vi "Capture.vi"(8 "error in (no error)":errorcluster, 9 "force_length":i8, 10 "capture_channel":u16, 11 "length":i32) -> (0 "error out":errorcluster, 3 "function return":i32)   [LabVIEW 2021, in "vmmsolib.lvlib"]
doc: "DLL_API int WINAPI Capture(int length, unsigned short capture_channel, char force_length);"
uses:
  vmmsolib.lvlib
  vmmso.dll
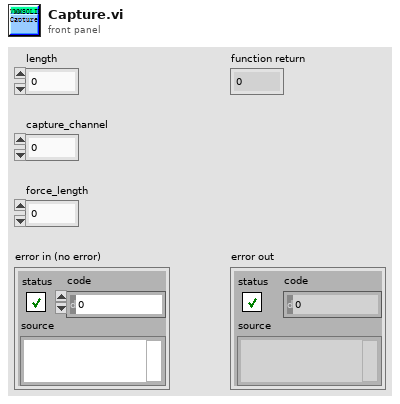
[diagram p1: front panel]
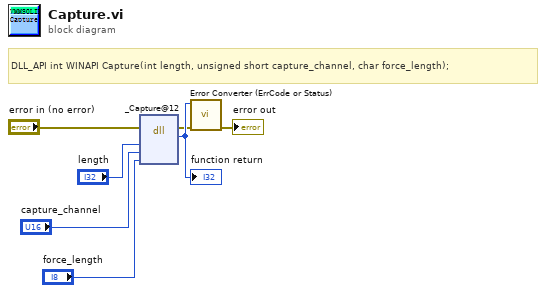
[diagram p0: block diagram]
diagram:
  # "DLL_API int WINAPI Capture(int length, unsigned short capture_channel, char force_length);"
  n1 = dll-call lib="D:/VmMsoSDK/demo-Labview/2021/vmmsolib/vmmso.*" fn="_Capture@12"(error in="error in (no error)", "length"="length", "capture_channel"="capture_channel", "force_length"="force_length") -> (error out=w2:errorcluster, w7:i32)  [unwired: 5 in, 1 out]
  "function return" <- w7
  n2 = call "Error Converter (ErrCode or Status).vi"("error in (no error)"=w2, "error code"=w7) -> ("error out"=→"error out":errorcluster)  [unwired: 9 in]
